vi "Initialization VI.vi"(8 "error in (no error)":errorcluster, 10 "Custom XML":string, 11 "Device Item Ref in":T1 format="%.0x") -> (0 "error out":errorcluster, 3 "Device Item Ref out":T1 format="%.0x")   [LabVIEW 2026, in "WebPage Addon System Explorer.lvlib"]
uses:
  WebPage Addon System Explorer.lvlib
  <vilib>/NI VeriStand/Custom Device API/Custom Device Item Ref.ctl
  Types/Main.Settings.ctl
  Types/Page Settings Action.ctl
  <vilib>/NI/NI VeriStand Custom Device Import and Export Tool/ImportExport.lvlib
  <vilib>/NI VeriStand/Custom Device Tools/Custom Device Utility Library/Custom Device Utility Library.lvlib
  <vilib>/NI VeriStand/Custom Device API/Custom Device API.lvlib
  NationalInstruments.VeriStand.SystemStorage
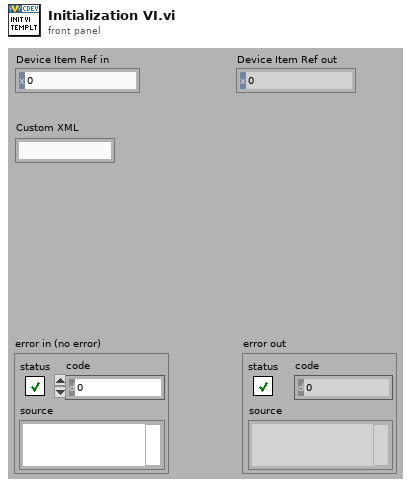
[diagram p1: front panel]
types:
  T1 = typedef "Custom Device API.lvlib/Custom Device Item Ref.ctl" = u64
  T2 = typedef "WebPage Addon System Explorer.lvlib/Page Settings Action.ctl" = enum16{"Get", "Set"}
  T3 = typedef "WebPage Addon System Explorer.lvlib/Main.Settings.ctl" = cluster{"Update Rate":dbl, "Hosted Port":u32, "gRPC Port":u32, "Hosted IP Address":string}
  T4 = typedef "Custom Device API.lvlib/Custom Device Pointer.ctl" = refnum<k24>
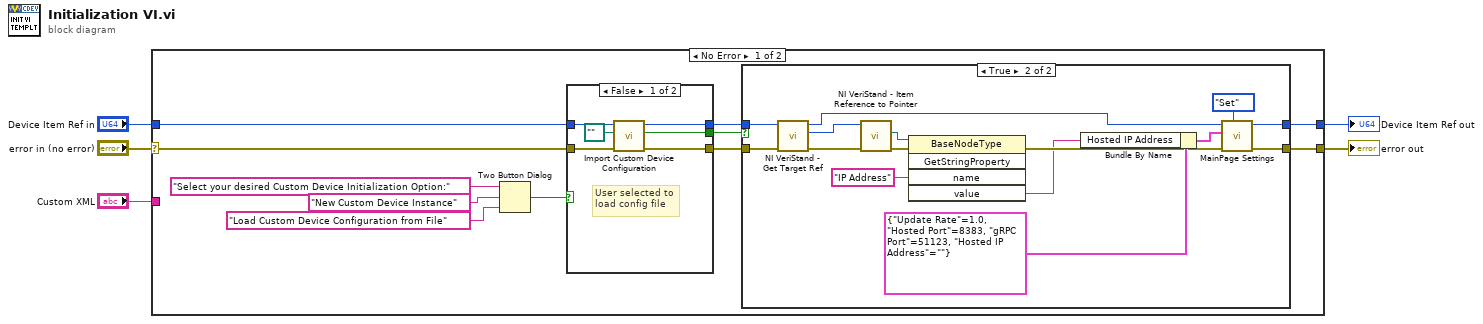
[diagram p0: block diagram]
diagram:
  n1 = case shown="No Error" "error in (no error)" {
    selector: "error in (no error)" -> [w11 w44]
    tunnel: [w7 w44] -> w5
    tunnel: [w6 w43] -> w3
    tunnel: "Device Item Ref in" -> [w12 w43]
    tunnel: "Custom XML" -> [_ _]
    frame No Error {
      n2 = Two Button Dialog(message="Select your desired Custom Device Initialization Option:", 1:"Load Custom Device Configuration from File" ("F button name (\"Cancel\")"), 2:"New Custom Device Instance" ("T button name (\"OK\")")) -> (T button?=w13:bool)
      n3 = case "New or Load" shown="False" w13 {
        selector: w13 -> [_ w40]
        tunnel: w12 -> [w39 w42]
        tunnel: [w38 w42] -> w10
        tunnel: w11 -> [w36 w41]
        tunnel: [w35 w41] -> w8
        tunnel: [w34 w40] -> w9
        frame False {
          # "User selected to\nload config file"
          n4 = call <vilib>:"Import Custom Device Configuration.vi"("error in (no error)"=w36, "Path"=path "", "NodeID"=w39) -> ("error out"=w35:errorcluster, "cancelled"=w34:bool, "NodeID out"=w38:u64)  [unwired: 6 in]
        }
        frame True {
          # "User selected new\ncustom device. Do\nnothing in this case\nand handle new\ngeneration in the\nnext case structure"
        }
      }
      n5 = case "Create New" shown="True" w9 {
        tunnel: w10 -> [w18 w29]
        tunnel: w8 -> [w17 w30]
        tunnel: [w17 w32] -> w7
        tunnel: [w18 w31] -> w6
        frame False {
        }
        frame True {
          n6 = call <vilib>:"NI VeriStand - Get Target Ref.vi"("error in"=w30, "Item Ref in"=w29) -> ("error out"=w24:errorcluster, "Target Ref"=w25:T1, "Item Ref out"=w26:T1)  [unwired: 6 in, 1 out]
          n7 = call <vilib>:"NI VeriStand - Item Reference to Pointer.vi"("error in (no error)"=w24, "Item Ref in"=w25) -> ("error out"=w21:errorcluster, "Node Pointer"=w23:T4)  [unwired: 6 in, 2 out]
          n8 = invoke class="BaseNodeType" method="GetStringProperty"(reference=w23, error in=w21, "name"="IP Address" ("Property Name")) -> (error out=w20:errorcluster, "value"=w19:string)  [unwired: 2 in, 3 out]
          n9 = Bundle By Name(cluster=T3 {"Update Rate"=1.0, "Hosted Port"=8383, "gRPC Port"=51123, "Hosted IP Address"=""}, "Hosted IP Address"=w19) -> (w27:T3)
          n10 = call "MainPage Settings.vi"("Action"=Page_Settings_Action."Set", "error in (no error)"=w20, "Settings In"=w27, "Item Ref in"=w26) -> ("error out"=w32:errorcluster, "Item Ref out"=w31:T1)  [unwired: 5 in, 1 out]
        }
      }
    }
    frame Error {
    }
  }
  "error out" <- w5
  "Device Item Ref out" <- w3
